vi "unix time 10ms.vi"() -> (0 "time stamp":timestamp, 1 "unix time (ms)":u64)   [LabVIEW 2019, in "Timers.lvlib"]
uses:
  Timers.lvlib
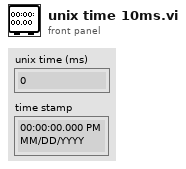
[diagram p1: front panel]
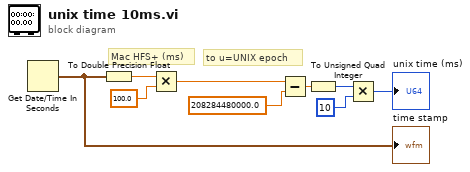
[diagram p0: block diagram]
diagram:
  # "to u=UNIX epoch"
  # "Mac HFS+ (ms)"
  n1 = Get Date/Time In Seconds() -> (seconds since 1Jan1904=w5:timestamp)
  "time stamp" <- w5
  n2 = To Double Precision Float(number=w5) -> (double precision float=w8:dbl)
  n3 = Multiply(x=w8, y=100.0) -> (x*y=w6:dbl)
  n4 = Subtract(x=w6, y=208284480000.0) -> (x-y=w4:dbl)
  n5 = To Unsigned Quad Integer(1:w4) -> (0:w2:u64)
  n6 = Multiply(x=w2, y=u64 10) -> (x*y=→"unix time (ms)":u64)
